vi "NI VeriStand - Pause Macro Player.vi"(8 "error in (no error)":errorcluster, 11 "MacroPlayer in":T1) -> (0 "error out":errorcluster, 3 "MacroPlayer out":T1)   [LabVIEW 2020, in "NI_VS MacroPlayerAPI.lvlib"]
doc: "Pauses the playback of a macro file. Use the Resume Macro Player VI to restart playback from the point where this VI pauses it."
uses:
  <vilib>/NI VeriStand/Execution/MacroPlayer/NI_VS MacroPlayerAPI.lvlib
  <vilib>/NI VeriStand/Execution/MacroPlayer/MacroPlayerAPI.ctl
  NationalInstruments.VeriStand.ClientAPI
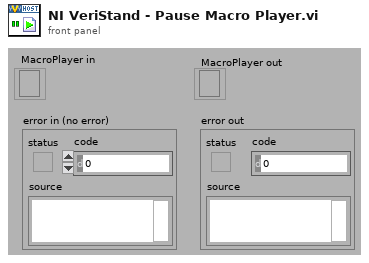
[diagram p1: front panel]
types:
  T1 = typedef "NI_VS MacroPlayerAPI.lvlib/MacroPlayerAPI.ctl" = refnum<k24>
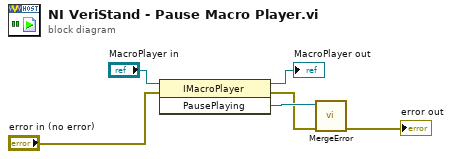
[diagram p0: block diagram]
diagram:
  n1 = invoke class="IMacroPlayer" method="PausePlaying"(reference="MacroPlayer in", error in="error in (no error)") -> (reference out=→"MacroPlayer out":T1, error out=w1:errorcluster, "PausePlaying"=w3:refnum<k24>)  [unwired: 1 in]
  n2 = call <vilib>:"MergeError.vi"("error in (no error)"=w1, "Error"=w3) -> ("error out"=→"error out":errorcluster)  [unwired: 9 out]
